vi "Periodic Tasks.vi"(8 "error in":errorcluster) -> ()   [LabVIEW 2013]
doc: "This VI runs in parallel to other tasks. It can contain as many user-defined periodic loops as you need. These can carry out PID or other sorts of timed response."
uses:
  <vilib>/Rock Robotics/SystemInterfaces/Utilities/FPGA_UtilitiesLED Source.ctl
  <vilib>/Rock Robotics/SystemInterfaces/Utilities/FPGA_UtilitiesLED State.ctl
  <vilib>/Rock Robotics/WPI/Solenoid/WPI_SolenoidValue.ctl
  <vilib>/Rock Robotics/WPI/Joystick/WPI_JoystickGetSetRefNum.vi
  Robot Global Data.vi
  <vilib>/Rock Robotics/WPI/Compressor/WPI_CompressorGetSetRefNum.vi
  <vilib>/Rock Robotics/WPI/RobotDrive/WPI_RobotDriveGetSetRefNum.vi
  <vilib>/Rock Robotics/WPI/Solenoid/WPI_SolenoidSetEnum.vi
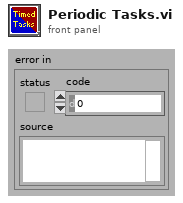
[diagram p1: front panel]
types:
  T1 = typedef "WPI_JoystickDevRef.ctl" = cluster{"Device":T2}
  T2 = typedef "WPI_JoystickDeviceEnum.ctl" = enum16{"USB 1", "USB 2", "USB 3", "USB 4", "Kinect 1", "Kinect 2"}
  T3 = typedef "WPI_RobotDriveDevRef.ctl" = cluster{"DevStatus":errorcluster, "Motors[]":T4[], "Square Inputs":bool, "Max Output":dbl, "Isochronous":bool}
  T4 = typedef "WPI_MotorControlDeviceRef.ctl" = cluster{"DeviceStatus":errorcluster, "Type":enum16{"PWM", "CAN"}, "PWM":cluster{"Digital Module":T5, "PWM Channel":T6, "DeadBand":T7}, "CAN":cluster{"Device Number":u8, "Control Mode":T8, "Semaphore":T9, "Max Vout":dbl}, "Invert":bool, "TransformRef":T10, "InvTransformRef":T10}
  T5 = typedef "FPGA_TypedefDigitalModule.ctl" = enum16{"Digital Module 1", "Digital Module 2"}
  T6 = typedef "FPGA_DIOPWMChannel.ctl" = enum8{"PWM 1", "PWM 2", "PWM 3", "PWM 4", "PWM 5", "PWM 6", "PWM 7", "PWM 8", "PWM 9", "PWM 10", "Invalid"}
  T7 = typedef "WPI_PWMDeadband.ctl" = cluster{"Name":string, "maxPositivePwm":i32, "minPositivePwm":i32, "centerPwm":i32, "maxNegativePwm":i32, "minNegativePwm":i32, "angularRange":u16}
  T8 = typedef "WPI_CANJaguar_ControlMode.ctl" = enum8{"Percent VBus", "Current", "Speed", "Position", "Voltage"}
  T9 = typedef "Semaphore RefNum" = refnum<k1>
  T10 = typedef "WPI_PWMTransform_ConPane.ctl" = refnum<vi>
  T11 = cluster{"JoystickDevRef":T1, "JoystickDevRef":T1, "JoystickDevRef":T1, "RobotDriveDevRef":T3}
  T12 = typedef "WPI_SolenoidValue.ctl" = enum16{"Off", "On", "Forward", "Reverse"}
  T13 = cluster{"A":bool, "B":bool, "X":bool, "Y":bool, "LB":bool, "RB":bool, "Back":bool, "Start":bool, "LS":bool, "RS":bool}
  T14 = typedef "WPI_DigitalInputDevRef.ctl" = cluster{"DevStatus":errorcluster, "DIO Channel":T15, "Digital Module":T5}
  T15 = typedef "FPGA_DIOChannel.ctl" = enum8{"DIO 1", "DIO 2", "DIO 3", "DIO 4", "DIO 5", "DIO 6", "DIO 7", "DIO 8", "DIO 9", "DIO 10", "DIO 11", "DIO 12", "DIO 13", "DIO 14", "Invalid"}
  T16 = typedef "WPI_SolenoidDevRef.ctl" = cluster{"DevStatus":errorcluster, "Solenoid Module":T17, "Forward Solenoid Channel":T18, "Reverse Solenoid Channel":T18}
  T17 = typedef "FPGA_TypedefSolenoidModule.ctl" = enum16{"Solenoid Module 1", "Solenoid Module 2"}
  T18 = typedef "WPI_SolenoidChannel.ctl" = enum8{"Solenoid 1", "Solenoid 2", "Solenoid 3", "Solenoid 4", "Solenoid 5", "Solenoid 6", "Solenoid 7", "Solenoid 8", "Invalid"}
  T19 = typedef "FPGA_UtilitiesLED State.ctl" = enum16{"Off", "On", "Toggle"}
  T20 = typedef "FPGA_UtilitiesLED Source.ctl" = enum16{"User LED", "FPGA LED"}
  T21 = typedef "WPI_AnalogChannelDevRef.ctl" = cluster{"DevStatus":errorcluster, "Analog Module":T22, "Analog Channel":T23}
  T22 = typedef "FPGA_TypedefAnalogModule.ctl" = enum16{"Analog Module 1", "Analog Module 2"}
  T23 = typedef "FPGA_AIChannel.ctl" = enum8{"AI 1", "AI 2", "AI 3", "AI 4", "AI 5", "AI 6", "AI 7", "AI 8", "Invalid"}
  T24 = typedef "WPI_CompressorDevRef.ctl" = cluster{"DevStatus":errorcluster, "DigitalInputDevRef":T14, "RelayDevRef":T25}
  T25 = typedef "WPI_RelayDevRef.ctl" = cluster{"DevStatus":errorcluster, "Relay Channel":T26, "Digital Module":T5, "Relay Direction":T27}
  T26 = typedef "FPGA_DIORelayChannel.ctl" = enum8{"Relay 1", "Relay 2", "Relay 3", "Relay 4", "Relay 5", "Relay 6", "Relay 7", "Relay 8", "Invalid"}
  T27 = typedef "WPI_RelayDirection.ctl" = enum16{"Both directions", "Forward only", "Reverse only"}
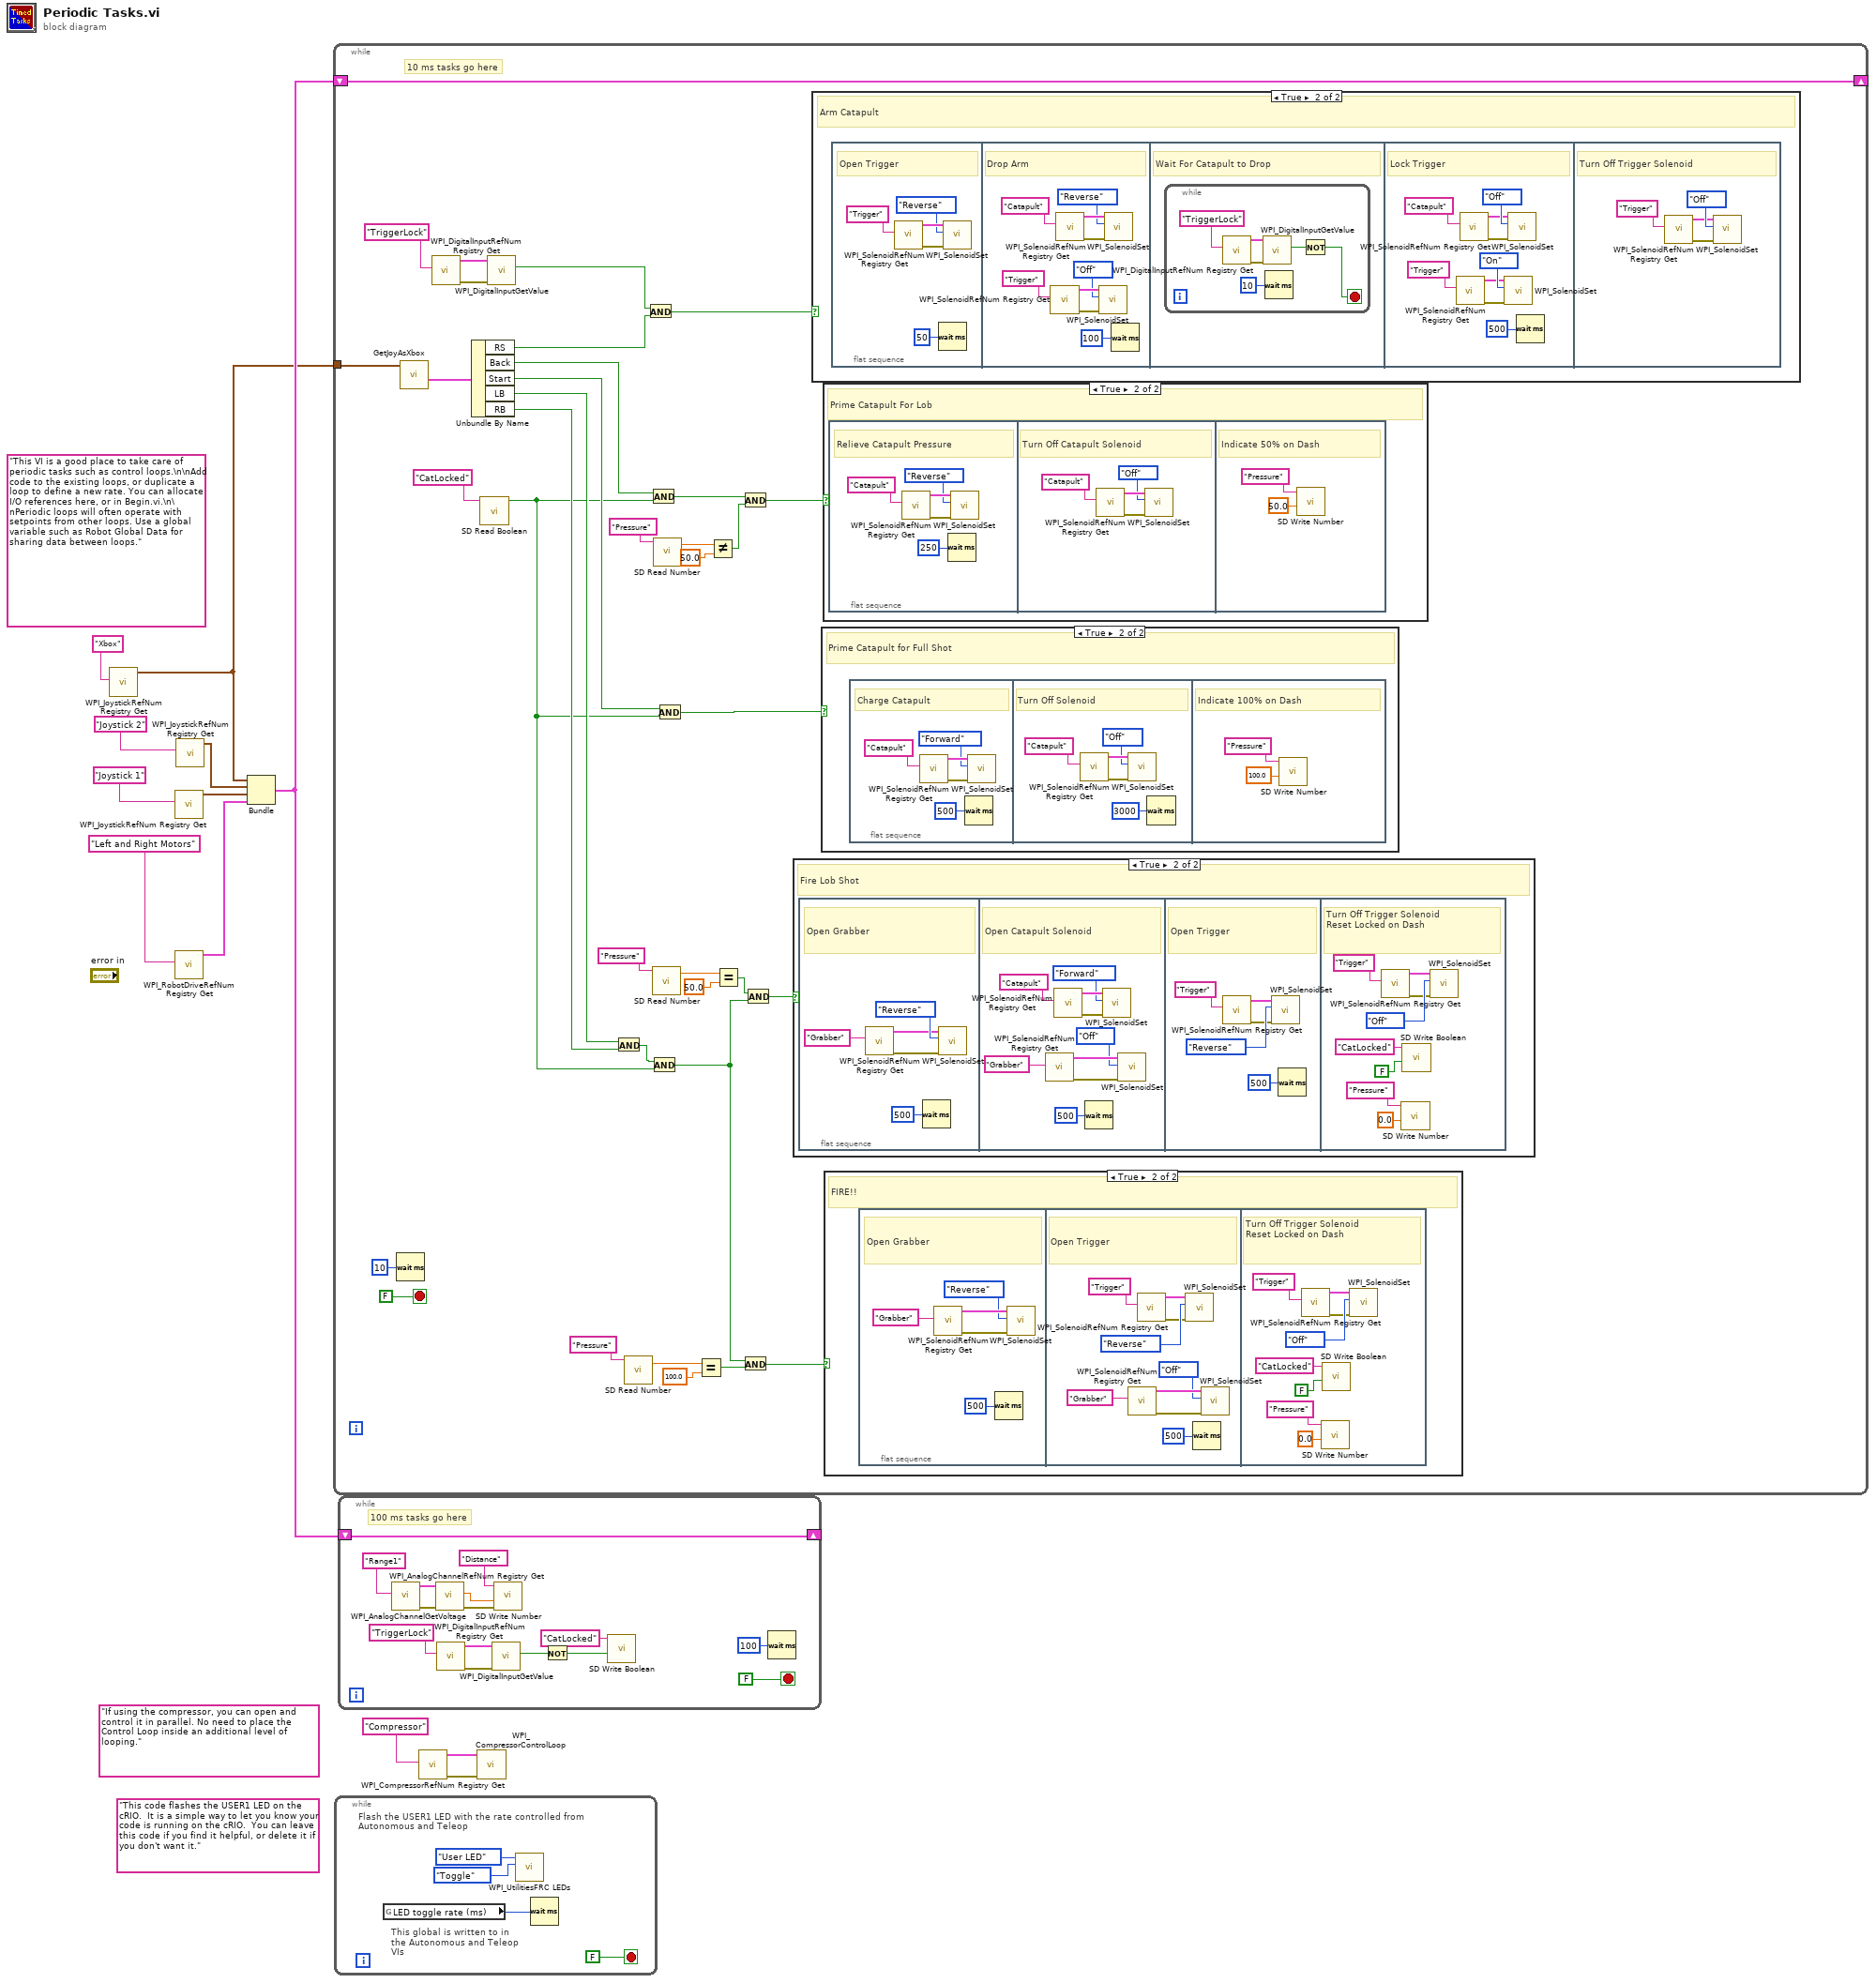
[diagram p0: block diagram]
diagram:
  (unwired) "If using the compressor, you can open and control it in parallel. No need to place the Control Loop inside an additional level of looping."
  (unwired) "This code flashes the USER1 LED on the cRIO.  It is a simple way to let you know your code is running on the cRIO.  You can leave this code if you find it helpful, or delete it if you don't want it."
  (unwired) "This VI is a good place to take care of periodic tasks such as control loops.\n\nAdd code to the existing loops, or duplicate a loop to define a new rate. You can allocate I/O references here, or in Begin.vi.\n\nPeriodic loops will often operate with setpoints from other loops. Use a global variable such as Robot Global Data for sharing data between loops."
  n1 = call <vilib>:"WPI_JoystickRefNum Registry Get.vi"("refnum name"="Xbox") -> ("JoystickDevRef"=w1:T1)  [unwired: 9 in, 1 out]
  n2 = call <vilib>:"WPI_JoystickRefNum Registry Get.vi"("refnum name"="Joystick 1") -> ("JoystickDevRef"=w10:T1)  [unwired: 1 in, 9 out]
  n3 = call <vilib>:"WPI_RobotDriveRefNum Registry Get.vi"("refnum name"="Left and Right Motors") -> ("RobotDriveDevRef"=w9:T3)  [unwired: 1 in, 9 out]
  n4 = call <vilib>:"WPI_JoystickRefNum Registry Get.vi"("refnum name"="Joystick 2") -> ("JoystickDevRef"=w7:T1)  [unwired: 1 in, 9 out]
  n5 = Bundle("JoystickDevRef"=w1, "JoystickDevRef"=w7, "JoystickDevRef"=w10, "RobotDriveDevRef"=w9) -> (w3:T11)  [unwired: 1 out]
  n6 = while {
    shift-right: [w46] -> _
    shift-left: w3 -> [w46]
    tunnel: w1 -> [w40]
    stop <- FALSE stop-if-true
    # "10 ms tasks go here"
    n7 = Wait (ms)(milliseconds to wait=u32 10) -> ()  [unwired: 1 out]
    n8 = call "GetJoyAsXbox.vi"("JoystickDevRef"=w40) -> ("Buttons"=w45:T13)  [unwired: 8 in, 2 out]
    n9 = call <vilib>:"WPI_DigitalInputRefNum Registry Get.vi"("refnum name"="TriggerLock") -> ("error out"=w43:errorcluster, "DigitalInputDevRef"=w42:T14)  [unwired: 9 in]
    n10 = Unbundle By Name(w45) -> ("RS"=w35:bool, "Back"=w33:bool, "Start"=w34:bool, "LB"=w38:bool, "RB"=w37:bool)
    n11 = call <vilib>:"SD Read Boolean.vi"("Name"="CatLocked") -> ("Boolean"=w25:bool)  [unwired: 8 in, 2 out]
    n12 = call <vilib>:"WPI_DigitalInputGetValue.vi"("error in (no error)"=w43, "DigitalInputDevRef"=w42) -> ("Value"=w13:bool)  [unwired: 7 in, 2 out]
    n13 = And(x=w38, y=w37) -> (x .and. y?=w26:bool)
    n14 = call <vilib>:"SD Read Number.vi"("Name"="Pressure") -> ("Numeric"=w28:dbl)  [unwired: 8 in, 2 out]
    n15 = And(x=w13, y=w35) -> (x .and. y?=w41:bool)
    n16 = And(x=w33, y=w25) -> (x .and. y?=w15:bool)
    n17 = And(x=w26, y=w25) -> (x .and. y?=w21:bool)
    n18 = call <vilib>:"SD Read Number.vi"("Name"="Pressure") -> ("Numeric"=w31:dbl)  [unwired: 8 in, 2 out]
    n19 = call <vilib>:"SD Read Number.vi"("Name"="Pressure") -> ("Numeric"=w18:dbl)  [unwired: 8 in, 2 out]
    n20 = And(x=w34, y=w25) -> (x .and. y?=w36:bool)
    n21 = Equal?(x=w28, y=100.0) -> (x = y?=w22:bool)
    n22 = Not Equal?(x=w18, y=50.0) -> (x != y?=w16:bool)
    n23 = Equal?(x=w31, y=50.0) -> (x = y?=w24:bool)
    n24 = And(x=w15, y=w16) -> (x .and. y?=w14:bool)
    n25 = And(x=w21, y=w22) -> (x .and. y?=w20:bool)
    n26 = And(x=w24, y=w21) -> (x .and. y?=w23:bool)
    n27 = case shown="True" w23 {
      frame False {
      }
      frame True {
        # "Fire Lob Shot"
        n28 = flat-sequence {
          frame #0 {
            # "Open Grabber"
            n29 = call <vilib>:"WPI_SolenoidRefNum Registry Get.vi"("refnum name"="Grabber") -> ("error out"=w51:errorcluster, "SolenoidDevRef"=w52:T16)  [unwired: 9 in]
            n30 = Wait (ms)(milliseconds to wait=u32 500) -> ()  [unwired: 1 out]
            n31 = call-poly <vilib>:"WPI_SolenoidSet.vi"("error in (no error)"=w51, "Value"=WPI_SolenoidValue."Reverse", "SolenoidDevRef"=w52) -> ()  [unwired: 7 in, 2 out]
          }
          frame #1 {
            # "Open Catapult Solenoid"
            n32 = call <vilib>:"WPI_SolenoidRefNum Registry Get.vi"("refnum name"="Grabber") -> ("error out"=w56:errorcluster, "SolenoidDevRef"=w55:T16)  [unwired: 9 in]
            n33 = call <vilib>:"WPI_SolenoidRefNum Registry Get.vi"("refnum name"="Catapult") -> ("error out"=w61:errorcluster, "SolenoidDevRef"=w60:T16)  [unwired: 9 in]
            n34 = Wait (ms)(milliseconds to wait=u32 500) -> ()  [unwired: 1 out]
            n35 = call-poly <vilib>:"WPI_SolenoidSet.vi"("error in (no error)"=w61, "Value"=WPI_SolenoidValue."Forward", "SolenoidDevRef"=w60) -> ()  [unwired: 7 in, 2 out]
            n36 = call-poly <vilib>:"WPI_SolenoidSet.vi"("error in (no error)"=w56, "Value"=WPI_SolenoidValue."Off", "SolenoidDevRef"=w55) -> ()  [unwired: 7 in, 2 out]
          }
          frame #2 {
            # "Open Trigger"
            n37 = call <vilib>:"WPI_SolenoidRefNum Registry Get.vi"("refnum name"="Trigger") -> ("error out"=w65:errorcluster, "SolenoidDevRef"=w64:T16)  [unwired: 9 in]
            n38 = call-poly <vilib>:"WPI_SolenoidSet.vi"("error in (no error)"=w65, "Value"=WPI_SolenoidValue."Reverse", "SolenoidDevRef"=w64) -> ()  [unwired: 7 in, 2 out]
            n39 = Wait (ms)(milliseconds to wait=u32 500) -> ()  [unwired: 1 out]
          }
          frame #3 {
            # "Turn Off Trigger Solenoid\nReset Locked on Dash"
            n40 = call <vilib>:"WPI_SolenoidRefNum Registry Get.vi"("refnum name"="Trigger") -> ("error out"=w73:errorcluster, "SolenoidDevRef"=w72:T16)  [unwired: 9 in]
            n41 = call <vilib>:"SD Write Number.vi"("Numeric"=0.0, "Name"="Pressure") -> ()  [unwired: 8 in, 2 out]
            n42 = call <vilib>:"SD Write Boolean.vi"("Boolean"=FALSE, "Name"="CatLocked") -> ()  [unwired: 8 in, 2 out]
            n43 = call-poly <vilib>:"WPI_SolenoidSet.vi"("error in (no error)"=w73, "Value"=WPI_SolenoidValue."Off", "SolenoidDevRef"=w72) -> ()  [unwired: 7 in, 2 out]
          }
        }
      }
    }
    n44 = case shown="True" w41 {
      frame False {
      }
      frame True {
        # "Arm Catapult"
        n45 = flat-sequence {
          frame #0 {
            # "Open Trigger"
            n46 = call <vilib>:"WPI_SolenoidRefNum Registry Get.vi"("refnum name"="Trigger") -> ("error out"=w124:errorcluster, "SolenoidDevRef"=w123:T16)  [unwired: 9 in]
            n47 = Wait (ms)(milliseconds to wait=u32 50) -> ()  [unwired: 1 out]
            n48 = call-poly <vilib>:"WPI_SolenoidSet.vi"("error in (no error)"=w124, "Value"=WPI_SolenoidValue."Reverse", "SolenoidDevRef"=w123) -> ()  [unwired: 7 in, 2 out]
          }
          frame #1 {
            # "Drop Arm"
            n49 = call <vilib>:"WPI_SolenoidRefNum Registry Get.vi"("refnum name"="Trigger") -> ("error out"=w133:errorcluster, "SolenoidDevRef"=w132:T16)  [unwired: 9 in]
            n50 = call <vilib>:"WPI_SolenoidRefNum Registry Get.vi"("refnum name"="Catapult") -> ("error out"=w129:errorcluster, "SolenoidDevRef"=w128:T16)  [unwired: 9 in]
            n51 = call-poly <vilib>:"WPI_SolenoidSet.vi"("error in (no error)"=w133, "Value"=WPI_SolenoidValue."Off", "SolenoidDevRef"=w132) -> ()  [unwired: 7 in, 2 out]
            n52 = call-poly <vilib>:"WPI_SolenoidSet.vi"("error in (no error)"=w129, "Value"=WPI_SolenoidValue."Reverse", "SolenoidDevRef"=w128) -> ()  [unwired: 7 in, 2 out]
            n53 = Wait (ms)(milliseconds to wait=u32 100) -> ()  [unwired: 1 out]
          }
          frame #2 {
            # "Wait For Catapult to Drop"
            n54 = while {
              stop <- w136 stop-if-true
              n55 = call <vilib>:"WPI_DigitalInputRefNum Registry Get.vi"("refnum name"="TriggerLock") -> ("error out"=w137:errorcluster, "DigitalInputDevRef"=w138:T14)  [unwired: 9 in]
              n56 = call <vilib>:"WPI_DigitalInputGetValue.vi"("error in (no error)"=w137, "DigitalInputDevRef"=w138) -> ("Value"=w139:bool)  [unwired: 7 in, 2 out]
              n57 = Wait (ms)(milliseconds to wait=u32 10) -> ()  [unwired: 1 out]
              n58 = Not(x=w139) -> (.not. x?=w136:bool)
            }
          }
          frame #3 {
            # "Lock Trigger"
            n59 = call <vilib>:"WPI_SolenoidRefNum Registry Get.vi"("refnum name"="Trigger") -> ("error out"=w142:errorcluster, "SolenoidDevRef"=w143:T16)  [unwired: 9 in]
            n60 = call <vilib>:"WPI_SolenoidRefNum Registry Get.vi"("refnum name"="Catapult") -> ("error out"=w146:errorcluster, "SolenoidDevRef"=w147:T16)  [unwired: 9 in]
            n61 = call-poly <vilib>:"WPI_SolenoidSet.vi"("error in (no error)"=w142, "Value"=WPI_SolenoidValue."On", "SolenoidDevRef"=w143) -> ()  [unwired: 7 in, 2 out]
            n62 = call-poly <vilib>:"WPI_SolenoidSet.vi"("error in (no error)"=w146, "Value"=WPI_SolenoidValue."Off", "SolenoidDevRef"=w147) -> ()  [unwired: 7 in, 2 out]
            n63 = Wait (ms)(milliseconds to wait=u32 500) -> ()  [unwired: 1 out]
          }
          frame #4 {
            # "Turn Off Trigger Solenoid"
            n64 = call <vilib>:"WPI_SolenoidRefNum Registry Get.vi"("refnum name"="Trigger") -> ("error out"=w151:errorcluster, "SolenoidDevRef"=w152:T16)  [unwired: 9 in]
            n65 = call-poly <vilib>:"WPI_SolenoidSet.vi"("error in (no error)"=w151, "Value"=WPI_SolenoidValue."Off", "SolenoidDevRef"=w152) -> ()  [unwired: 7 in, 2 out]
          }
        }
      }
    }
    n66 = case shown="True" w36 {
      frame False {
      }
      frame True {
        # "Prime Catapult for Full Shot"
        n67 = flat-sequence {
          frame #0 {
            # "Charge Catapult"
            n68 = call <vilib>:"WPI_SolenoidRefNum Registry Get.vi"("refnum name"="Catapult") -> ("error out"=w112:errorcluster, "SolenoidDevRef"=w111:T16)  [unwired: 9 in]
            n69 = Wait (ms)(milliseconds to wait=u32 500) -> ()  [unwired: 1 out]
            n70 = call-poly <vilib>:"WPI_SolenoidSet.vi"("error in (no error)"=w112, "Value"=WPI_SolenoidValue."Forward", "SolenoidDevRef"=w111) -> ()  [unwired: 7 in, 2 out]
          }
          frame #1 {
            # "Turn Off Solenoid"
            n71 = call <vilib>:"WPI_SolenoidRefNum Registry Get.vi"("refnum name"="Catapult") -> ("error out"=w117:errorcluster, "SolenoidDevRef"=w116:T16)  [unwired: 9 in]
            n72 = call-poly <vilib>:"WPI_SolenoidSet.vi"("error in (no error)"=w117, "Value"=WPI_SolenoidValue."Off", "SolenoidDevRef"=w116) -> ()  [unwired: 7 in, 2 out]
            n73 = Wait (ms)(milliseconds to wait=u32 3000) -> ()  [unwired: 1 out]
          }
          frame #2 {
            # "Indicate 100% on Dash"
            n74 = call <vilib>:"SD Write Number.vi"("Numeric"=100.0, "Name"="Pressure") -> ()  [unwired: 8 in, 2 out]
          }
        }
      }
    }
    n75 = case shown="True" w14 {
      frame False {
      }
      frame True {
        # "Prime Catapult For Lob"
        n76 = flat-sequence {
          frame #0 {
            # "Relieve Catapult Pressure"
            n77 = call <vilib>:"WPI_SolenoidRefNum Registry Get.vi"("refnum name"="Catapult") -> ("error out"=w101:errorcluster, "SolenoidDevRef"=w100:T16)  [unwired: 9 in]
            n78 = Wait (ms)(milliseconds to wait=u32 250) -> ()  [unwired: 1 out]
            n79 = call-poly <vilib>:"WPI_SolenoidSet.vi"("error in (no error)"=w101, "Value"=WPI_SolenoidValue."Reverse", "SolenoidDevRef"=w100) -> ()  [unwired: 7 in, 2 out]
          }
          frame #1 {
            # "Turn Off Catapult Solenoid"
            n80 = call <vilib>:"WPI_SolenoidRefNum Registry Get.vi"("refnum name"="Catapult") -> ("error out"=w105:errorcluster, "SolenoidDevRef"=w104:T16)  [unwired: 9 in]
            n81 = call-poly <vilib>:"WPI_SolenoidSet.vi"("error in (no error)"=w105, "Value"=WPI_SolenoidValue."Off", "SolenoidDevRef"=w104) -> ()  [unwired: 7 in, 2 out]
          }
          frame #2 {
            # "Indicate 50% on Dash"
            n82 = call <vilib>:"SD Write Number.vi"("Numeric"=50.0, "Name"="Pressure") -> ()  [unwired: 8 in, 2 out]
          }
        }
      }
    }
    n83 = case shown="True" w20 {
      frame False {
      }
      frame True {
        # "FIRE!!"
        n84 = flat-sequence {
          frame #0 {
            # "Open Grabber"
            n85 = call <vilib>:"WPI_SolenoidRefNum Registry Get.vi"("refnum name"="Grabber") -> ("error out"=w79:errorcluster, "SolenoidDevRef"=w78:T16)  [unwired: 9 in]
            n86 = Wait (ms)(milliseconds to wait=u32 500) -> ()  [unwired: 1 out]
            n87 = call-poly <vilib>:"WPI_SolenoidSet.vi"("error in (no error)"=w79, "Value"=WPI_SolenoidValue."Reverse", "SolenoidDevRef"=w78) -> ()  [unwired: 7 in, 2 out]
          }
          frame #1 {
            # "Open Trigger"
            n88 = call <vilib>:"WPI_SolenoidRefNum Registry Get.vi"("refnum name"="Grabber") -> ("error out"=w83:errorcluster, "SolenoidDevRef"=w82:T16)  [unwired: 9 in]
            n89 = call <vilib>:"WPI_SolenoidRefNum Registry Get.vi"("refnum name"="Trigger") -> ("error out"=w87:errorcluster, "SolenoidDevRef"=w86:T16)  [unwired: 9 in]
            n90 = call-poly <vilib>:"WPI_SolenoidSet.vi"("error in (no error)"=w87, "Value"=WPI_SolenoidValue."Reverse", "SolenoidDevRef"=w86) -> ()  [unwired: 7 in, 2 out]
            n91 = Wait (ms)(milliseconds to wait=u32 500) -> ()  [unwired: 1 out]
            n92 = call-poly <vilib>:"WPI_SolenoidSet.vi"("error in (no error)"=w83, "Value"=WPI_SolenoidValue."Off", "SolenoidDevRef"=w82) -> ()  [unwired: 7 in, 2 out]
          }
          frame #2 {
            # "Turn Off Trigger Solenoid\nReset Locked on Dash"
            n93 = call <vilib>:"WPI_SolenoidRefNum Registry Get.vi"("refnum name"="Trigger") -> ("error out"=w95:errorcluster, "SolenoidDevRef"=w94:T16)  [unwired: 9 in]
            n94 = call <vilib>:"SD Write Number.vi"("Numeric"=0.0, "Name"="Pressure") -> ()  [unwired: 8 in, 2 out]
            n95 = call <vilib>:"SD Write Boolean.vi"("Boolean"=FALSE, "Name"="CatLocked") -> ()  [unwired: 8 in, 2 out]
            n96 = call-poly <vilib>:"WPI_SolenoidSet.vi"("error in (no error)"=w95, "Value"=WPI_SolenoidValue."Off", "SolenoidDevRef"=w94) -> ()  [unwired: 7 in, 2 out]
          }
        }
      }
    }
  }
  n97 = while {
    stop <- FALSE stop-if-true
    # "This global is written to in the Autonomous and Teleop VIs"
    # "Flash the USER1 LED with the rate controlled from Autonomous and Teleop"
    n98 = global read "Robot Global Data.vi" "LED toggle rate (ms)"() -> (w154:u32)
    n99 = call <vilib>:"WPI_UtilitiesFRC LEDs.vi"("State"=FPGA_UtilitiesLED_State."Toggle", "LED Type"=FPGA_UtilitiesLED_Source."User LED") -> ()  [unwired: 1 in, 9 out]
    n100 = Wait (ms)(milliseconds to wait=w154) -> ()  [unwired: 1 out]
  }
  n101 = while {
    shift-right: [w170] -> _
    shift-left: w3 -> [w170]
    stop <- FALSE stop-if-true
    # "100 ms tasks go here"
    n102 = call <vilib>:"WPI_AnalogChannelRefNum Registry Get.vi"("refnum name"="Range1") -> ("error out"=w168:errorcluster, "AIDeviceRef"=w167:T21)  [unwired: 9 in]
    n103 = call <vilib>:"WPI_AnalogChannelGetVoltage.vi"("error in (no error)"=w168, "AIDeviceRef"=w167) -> ("error out"=w166:errorcluster, "Voltage"=w164:dbl)  [unwired: 7 in, 1 out]
    n104 = call <vilib>:"WPI_DigitalInputRefNum Registry Get.vi"("refnum name"="TriggerLock") -> ("error out"=w161:errorcluster, "DigitalInputDevRef"=w162:T14)  [unwired: 9 in]
    n105 = call <vilib>:"WPI_DigitalInputGetValue.vi"("error in (no error)"=w161, "DigitalInputDevRef"=w162) -> ("Value"=w159:bool)  [unwired: 7 in, 2 out]
    n106 = call <vilib>:"SD Write Number.vi"("error in"=w166, "Numeric"=w164, "Name"="Distance") -> ()  [unwired: 7 in, 2 out]
    n107 = Not(x=w159) -> (.not. x?=w158:bool)
    n108 = call <vilib>:"SD Write Boolean.vi"("Boolean"=w158, "Name"="CatLocked") -> ()  [unwired: 8 in, 2 out]
    n109 = Wait (ms)(milliseconds to wait=u32 100) -> ()  [unwired: 1 out]
  }
  n110 = call <vilib>:"WPI_CompressorRefNum Registry Get.vi"("refnum name"="Compressor") -> ("error out"=w5:errorcluster, "CompressorDevRef"=w4:T24)  [unwired: 9 in]
  n111 = call <vilib>:"WPI_CompressorControlLoop.vi"("error in (no error)"=w5, "CompressorDevRef"=w4) -> ()  [unwired: 10 in]
